vi "WinCOLORREF.vi"() -> ()   [LabVIEW 2023]
doc: "If input is black, then output will be blue. Otherwise, output will be green.\n\nFor information on the data types used for the DLL function, right-click on the Call Library Function node and choose Configure."
uses:
  CLF_Example.dll
panel:
  out "output":u32(colorbox)
  in  "input":u32(colorbox)
  # "See the block diagram for more information."
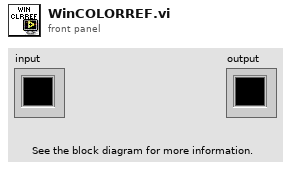
[diagram p1: front panel]
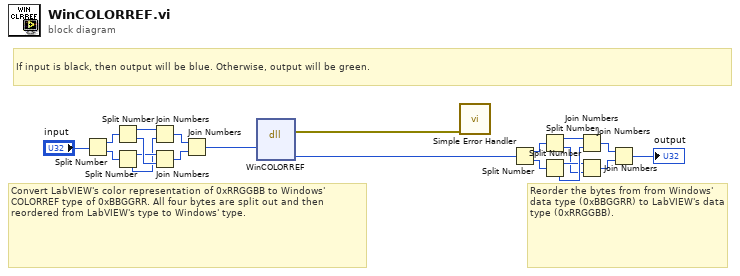
[diagram p0: block diagram]
diagram:
  # "If input is black, then output will be blue. Otherwise, output will be green."
  # "Reorder the bytes from from Windows' data type (0xBBGGRR) to LabVIEW's data type (0xRRGGBB)."
  # "Convert LabVIEW's color representation of 0xRRGGBB to Windows' COLORREF type of 0xBBGGRR. All four bytes are split out and then reordered from LabVIEW's type to Windows' type."
  n1 = Split Number(x="input") -> (hi(x)=w20:u16, lo(x)=w19:u16)
  n2 = Split Number(x=w20) -> (hi(x)=w18:u8, lo(x)=w17:u8)
  n3 = Split Number(x=w19) -> (hi(x)=w16:u8, lo(x)=w15:u8)
  n4 = Join Numbers(hi=w18, lo=w15) -> ((hi.lo)=w14:u16)
  n5 = Join Numbers(hi=w16, lo=w17) -> ((hi.lo)=w13:u16)
  n6 = Join Numbers(hi=w14, lo=w13) -> ((hi.lo)=w12:u32)
  n7 = dll-call lib="c:/dev/_r/4/eng/lv-core/lvpostprocessingd/lv_mc_x86_64/dist_i386/examples/Connectivity/Libraries and Executables/DLL Calling VIs/CLF_Example**.*" fn="WinCOLORREF"("input"=w12) -> (error out=w1:errorcluster, "output"=w3:u32)  [unwired: 4 in, 3 out]
  n8 = call <vilib>:"Simple Error Handler.vi"("error in (no error)"=w1) -> ()  [unwired: 4 in, 5 out]
  n9 = Split Number(x=w3) -> (hi(x)=w4:u16, lo(x)=w5:u16)
  n10 = Split Number(x=w4) -> (hi(x)=w6:u8, lo(x)=w7:u8)
  n11 = Split Number(x=w5) -> (hi(x)=w8:u8, lo(x)=w9:u8)
  n12 = Join Numbers(hi=w6, lo=w9) -> ((hi.lo)=w10:u16)
  n13 = Join Numbers(hi=w8, lo=w7) -> ((hi.lo)=w11:u16)
  n14 = Join Numbers(hi=w10, lo=w11) -> ((hi.lo)=→"output":u32)
